vi "Read All Nested Queues.vi"(8 "error in (no error)":errorcluster, 11 "Mag Lab Measure Base in":refnum<class "Mag Lab Measure Base.lvclass">) -> (0 "error out":errorcluster, 1 "Array of Queues":refnum<class "Message Enqueuer.lvclass">[](array[class]), 2 "names":string[](array[string]), 3 "Mag Lab Measure Base out":refnum<class "Mag Lab Measure Base.lvclass">)   [LabVIEW 2015, in "Mag Lab Measure Base.lvclass"]
uses:
  Mag Lab Measure Base.lvclass
  <vilib>/ActorFramework/Message Enqueuer/Message Enqueuer.lvclass
  Mag Lab Measure Base.lvclass/Mag Lab Measure Base.ctl
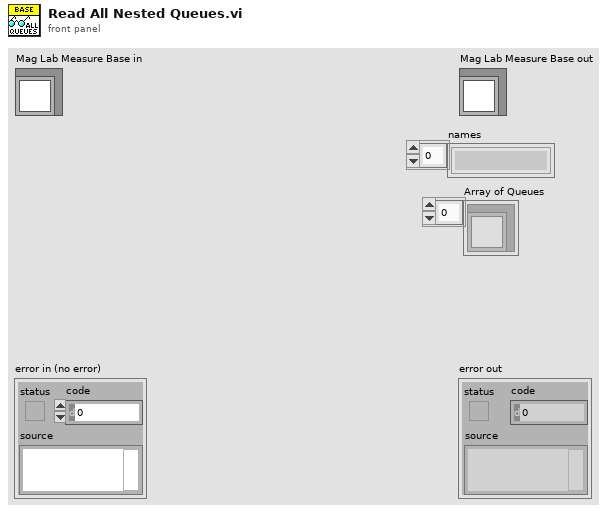
[diagram p1: front panel]
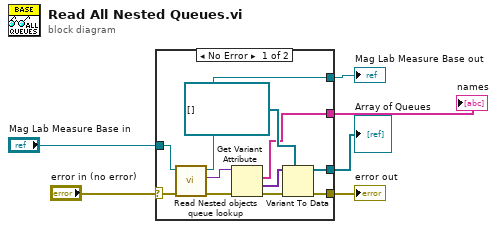
[diagram p0: block diagram]
diagram:
  n1 = case shown="No Error" "error in (no error)" {
    selector: "error in (no error)" -> [w11 w19]
    tunnel: [w9 w19] -> w5
    tunnel: [w14 w18] -> w3
    tunnel: "Mag Lab Measure Base in" -> [w17 w18]
    tunnel: [w8 _] -> w2
    tunnel: [w7 _] -> w1
    frame No Error {
      n2 = call "Read Nested objects queue lookup.vi"("error in (no error)"=w11, "Mag Lab Measure Base in"=w17) -> ("error out"=w10:errorcluster, "Nested objects queue lookup"=w13:variant, "Mag Lab Measure Base out"=w14:refnum<class "Mag Lab Measure Base.lvclass">)  [unwired: 7 in]
      n3 = Get Variant Attribute(Variant=w13, error in=w10) -> (names=w7:string[], values=w15:variant[], error out=w12:errorcluster)  [unwired: 2 in, 1 out]
      n4 = Variant To Data(error in=w12, type=refnum<class "Message Enqueuer.lvclass">[] [], Variant=w15) -> (data=w8:refnum<class "Message Enqueuer.lvclass">[], error out=w9:errorcluster)
    }
    frame Error {
    }
  }
  "error out" <- w5
  "Mag Lab Measure Base out" <- w3
  "Array of Queues" <- w2
  "names" <- w1
